vi "escribeEnTabla.vi"(9 "parametros":string[](array[string]), 10 "col":i32=2, 11 "tabla in":string[][](array[string])) -> (3 "tabla out":string[][](array[string]))   [LabVIEW 2019, in "Prueba.lvclass"]
uses:
  Prueba.lvclass
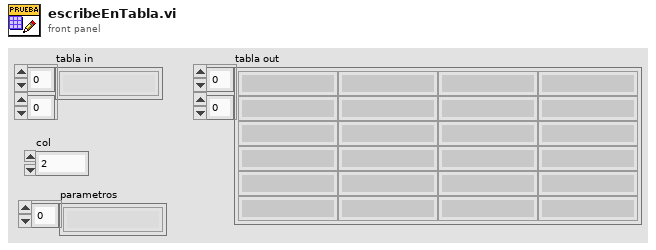
[diagram p1: front panel]
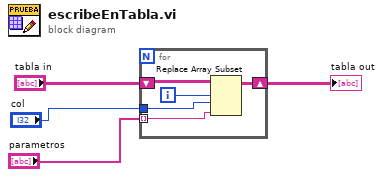
[diagram p0: block diagram]
diagram:
  n1 = for {
    shift-right: [w8] -> w4
    shift-left: "tabla in" -> [w9]
    tunnel: "parametros" -> [w6] mode=indexing
    tunnel: "col" -> [w5]
    i -> [w7]
    n2 = Replace Array Subset(array=w9, new element=w6, index (row)=w7, index (col)=w5) -> (w8:string[][])
  }
  "tabla out" <- w4
